vi "relative_angle.vi"(11 "y angle":dbl[](array[numeric])) -> (3 "Array":i32[][](array[numeric]))   [LabVIEW 2015]
panel:
  out "Array 2":dbl[](array[numeric])
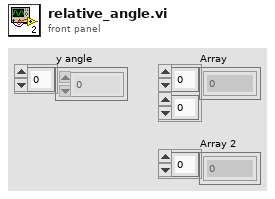
[diagram p1: front panel]
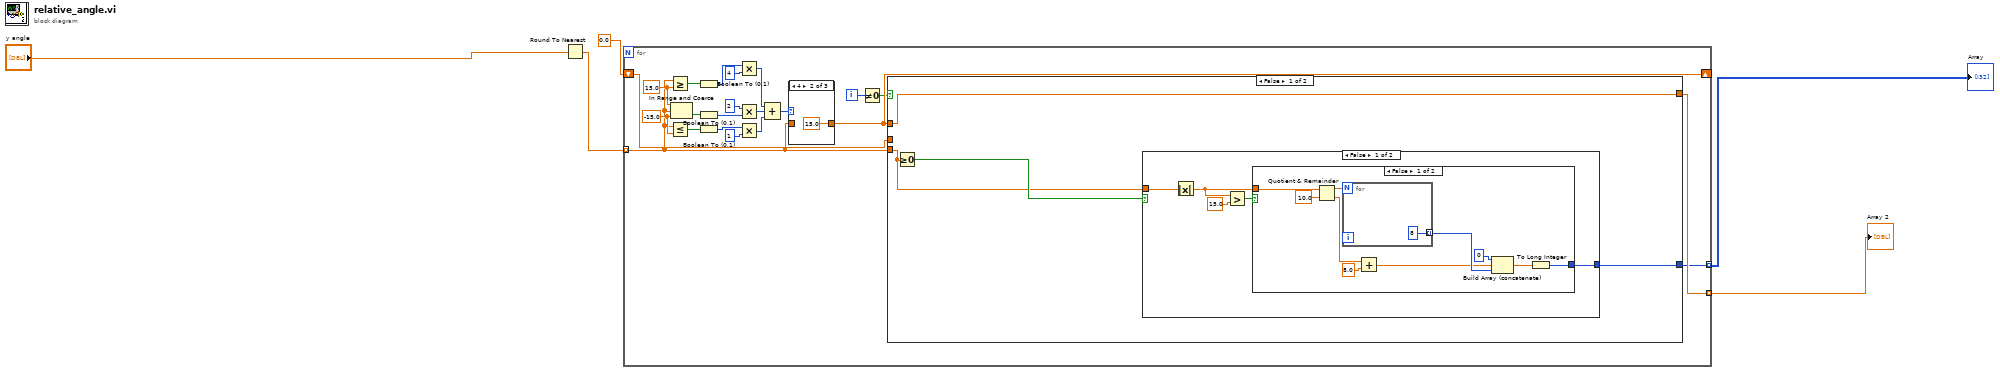
[diagram p0: block diagram]
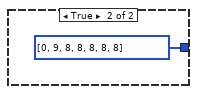
[diagram p2: hidden frame]
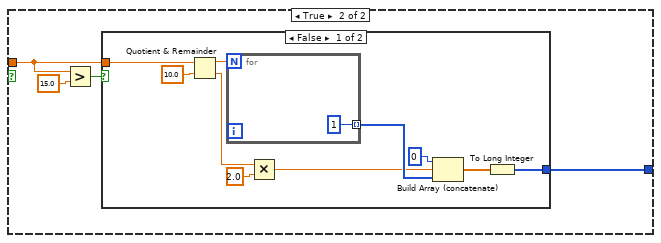
[diagram p3: hidden frame]
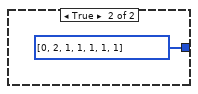
[diagram p4: hidden frame]
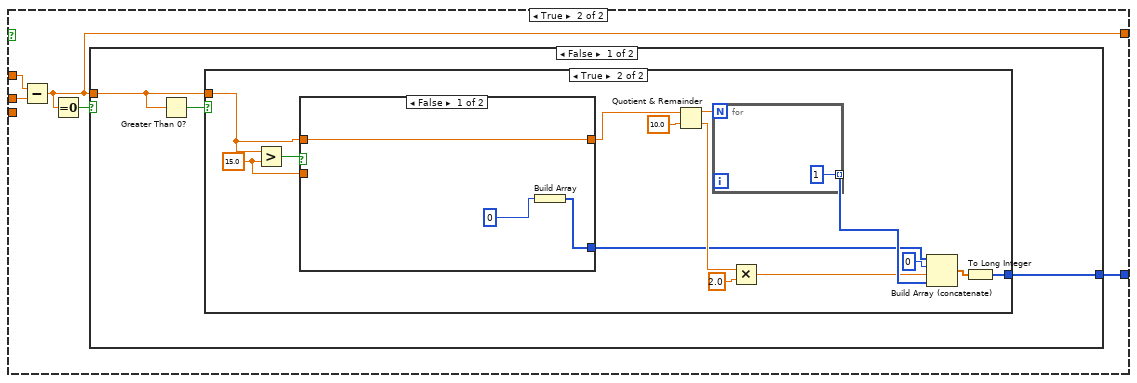
[diagram p5: hidden frame]
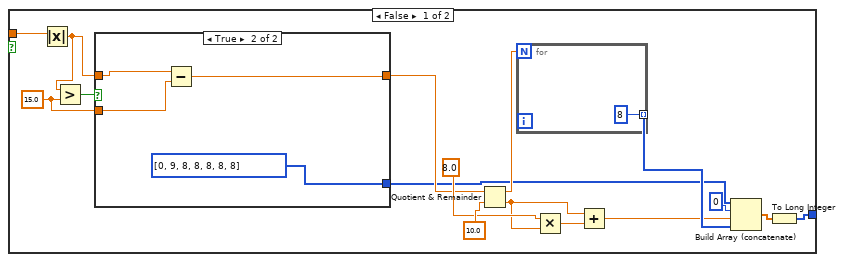
[diagram p6: hidden frame]
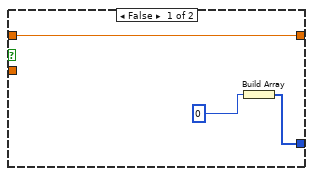
[diagram p7: hidden frame]
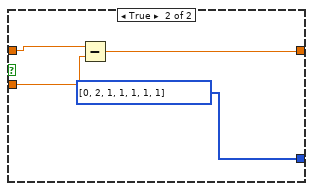
[diagram p8: hidden frame]
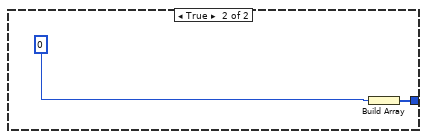
[diagram p9: hidden frame]
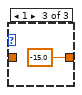
[diagram p11: hidden frame]
diagram:
  n1 = Round To Nearest(number="y angle") -> (nearest integer value=w2:dbl[])
  n2 = for {
    tunnel: w2 -> [w6] mode=indexing
    shift-right: [w11] -> _
    shift-left: 0.0 -> [w12]
    tunnel: [w10] -> w1 mode=indexing
    tunnel: [w9] -> w4 mode=indexing
    i -> [w8]
    w26 = -15.0 ("lower limit")
    w27 = 15.0 ("upper limit")
    n3 = Greater Or Equal?(x=w6, y=w27) -> (x >= y?=w24:bool)
    n4 = Less Or Equal?(x=w6, y=w26) -> (x <= y?=w23:bool)
    n5 = In Range and Coerce(upper limit=w27, x=w6, lower limit=w26) -> (In Range?=w25:bool)  [unwired: 1 out]
    n6 = Boolean To (0,1)(Boolean=w24) -> (0, 1=w22:i16)
    n7 = Boolean To (0,1)(Boolean=w25) -> (0, 1=w20:i16)
    n8 = Boolean To (0,1)(Boolean=w23) -> (0, 1=w18:i16)
    n9 = Multiply(x=w22, y=i16 4) -> (x*y=w16:i16)
    n10 = Multiply(x=i16 2, y=w20) -> (x*y=w15:i16)
    n11 = Multiply(x=w18, y=i16 1) -> (x*y=w14:i16)
    n12 = Compound Arithmetic op=ADD(w16, w15, w14) -> (w13:i16)
    n13 = case shown="4" w13 {
      tunnel: w6 -> [w121 _ _]
      tunnel: [w121 15.0 -15.0] -> w11
      frame 2, Default {
      }
      frame 4 {
      }
      frame 1 {
      }
    }
    n14 = Not Equal To 0?(x=w8) -> (x != 0?=w7:bool)
    n15 = case shown="False" w7 {
      tunnel: w12 -> [_ w69]
      tunnel: w11 -> [w29 w67]
      tunnel: [w29 w66] -> w10
      tunnel: [w30 w65] -> w9
      tunnel: w6 -> [w28 _]
      frame False {
        n16 = Greater Or Equal To 0?(x=w28) -> (x >= 0?=w31:bool)
        n17 = case shown="False" w31 {
          tunnel: [w33 w50] -> w30
          tunnel: w28 -> [w32 w49]
          frame False {
            n18 = Absolute Value(x=w32) -> (abs(x)=w34:dbl)
            n19 = Greater?(x=w34, y=15.0) -> (0:w35:bool)
            n20 = case shown="False" w35 {
              tunnel: [w43 i32[] [0, 9, 8, 8, 8, 8, 8]] -> w33
              tunnel: w34 -> [w37 _]
              frame False {
                n21 = Quotient & Remainder(x=w37, y=10.0) -> (x-y*floor(x/y)=w46:dbl, floor(x/y)=w38:dbl)
                n22 = for {
                  N: w46 -> [_]
                  tunnel: [8] -> w45 mode=indexing
                }
                n23 = Add(x=w38, y=8.0) -> (x+y=w40:dbl)
                n24 = Build Array (concatenate)(0, w40, w45) -> (w44:dbl[])
                n25 = To Long Integer(number=w44) -> (32bit integer=w43:i32[])
              }
              frame True {
              }
            }
          }
          frame True {
            n26 = Greater?(x=w49, y=15.0) -> (0:w51:bool)
            n27 = case shown="False" w51 {
              tunnel: [w59 i32[] [0, 2, 1, 1, 1, 1, 1]] -> w50
              tunnel: w49 -> [w53 _]
              frame False {
                n28 = Quotient & Remainder(x=w53, y=10.0) -> (x-y*floor(x/y)=w62:dbl, floor(x/y)=w54:dbl)
                n29 = for {
                  N: w62 -> [_]
                  tunnel: [1] -> w61 mode=indexing
                }
                n30 = Multiply(x=w54, y=2.0) -> (x*y=w56:dbl)
                n31 = Build Array (concatenate)(0, w56, w61) -> (w60:dbl[])
                n32 = To Long Integer(number=w60) -> (32bit integer=w59:i32[])
              }
              frame True {
              }
            }
          }
        }
      }
      frame True {
        n33 = Subtract(x=w67, y=w69) -> (x-y=w66:dbl)
        n34 = Equal To 0?(x=w66) -> (x = 0?=w68:bool)
        n35 = case shown="False" w68 {
          tunnel: w66 -> [w70 _]
          tunnel: [w71 w119] -> w65
          frame False {
            n36 = Greater Than 0?(x=w70) -> (x > 0?=w72:bool)
            n37 = case shown="True" w72 {
              tunnel: [w83 w102] -> w71
              tunnel: w70 -> [w78 w100]
              frame False {
                w73 = 15.0 ("y")
                n38 = Absolute Value(x=w78) -> (abs(x)=w75:dbl)
                n39 = Greater?(x=w75, y=w73) -> (0:w74:bool)
                n40 = case shown="True" w74 {
                  tunnel: w75 -> [w91 w95]
                  tunnel: [w91 w94] -> w77
                  tunnel: [w89 i32[] [0, 9, 8, 8, 8, 8, 8]] -> w76
                  tunnel: w73 -> [_ w92]
                  frame False {
                    n41 = Build Array(0) -> (w89:i32[])
                  }
                  frame True {
                    n42 = Subtract(x=w95, y=w92) -> (x-y=w94:dbl)
                  }
                }
                n43 = Quotient & Remainder(x=w77, y=10.0) -> (x-y*floor(x/y)=w82:dbl, floor(x/y)=w80:dbl)
                n44 = for {
                  N: w82 -> [_]
                  tunnel: [8] -> w88 mode=indexing
                }
                n45 = Multiply(x=8.0, y=w80) -> (x*y=w79:dbl)
                n46 = Add(x=w80, y=w79) -> (x+y=w84:dbl)
                n47 = Build Array (concatenate)(w76, 0, w84, w88) -> (w87:dbl[])
                n48 = To Long Integer(number=w87) -> (32bit integer=w83:i32[])
              }
              frame True {
                w98 = 15.0 ("y")
                n49 = Greater?(x=w100, y=w98) -> (0:w101:bool)
                n50 = case shown="False" w101 {
                  tunnel: w100 -> [w113 w117]
                  tunnel: [w113 w115] -> w99
                  tunnel: w98 -> [_ w116]
                  tunnel: [w111 i32[] [0, 2, 1, 1, 1, 1, 1]] -> w97
                  frame False {
                    n51 = Build Array(0) -> (w111:i32[])
                  }
                  frame True {
                    n52 = Subtract(x=w117, y=w116) -> (x-y=w115:dbl)
                  }
                }
                n53 = Quotient & Remainder(x=w99, y=10.0) -> (x-y*floor(x/y)=w110:dbl, floor(x/y)=w103:dbl)
                n54 = for {
                  N: w110 -> [_]
                  tunnel: [1] -> w109 mode=indexing
                }
                n55 = Multiply(x=w103, y=2.0) -> (x*y=w105:dbl)
                n56 = Build Array (concatenate)(w97, 0, w105, w109) -> (w108:dbl[])
                n57 = To Long Integer(number=w108) -> (32bit integer=w102:i32[])
              }
            }
          }
          frame True {
            n58 = Build Array(0) -> (w119:i32[])
          }
        }
      }
    }
  }
  "Array" <- w4
  "Array 2" <- w1
